vi "Read Project Path.vi"(8 "error in (no error)":errorcluster, 11 "Session in":refnum<class "Plugin Session.lvclass">) -> (0 "error out":errorcluster, 2 "Project Path":path, 3 "Session out":refnum<class "Plugin Session.lvclass">)   [LabVIEW 2021, in "InstrumentStudio Plugin SDK.lvlib" / "Plugin Session.lvclass"]
doc: "Call this VI to retrieve the absolute path of the InstrumentStudio project file on disk"
uses:
  Plugin Session.lvclass
  Plugin Session.lvclass/Plugin Session.ctl
  Read Session Id.vi
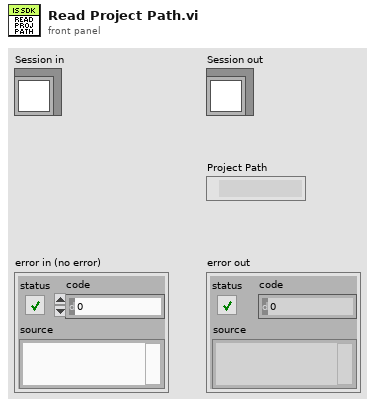
[diagram p1: front panel]
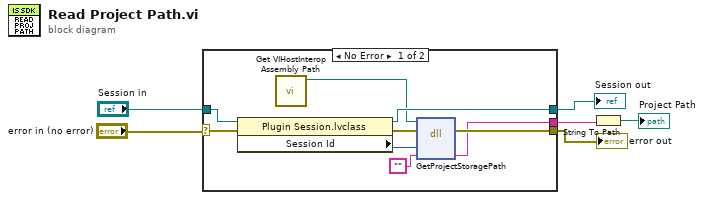
[diagram p0: block diagram]
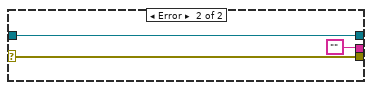
[diagram p2: hidden frame]
diagram:
  n1 = case shown="No Error" "error in (no error)" {
    selector: "error in (no error)" -> [w10 w17]
    tunnel: [w12 w17] -> w6
    tunnel: "Session in" -> [w11 w18]
    tunnel: [w9 w18] -> w3
    tunnel: [w8 ""] -> w2
    frame No Error {
      n2 = property class="Plugin Session.lvclass"(reference=w11, error in=w10) -> (reference out=w9:refnum<class "Plugin Session.lvclass">, error out=w15:errorcluster, "Session Id"=w14:u64)
      n3 = call "Get VIHostInterop Assembly Path.vi"() -> ("VIHost.Interop Assembly"=w7:path)  [unwired: 11 in]
      n4 = dll-call lib="C:/ASW/Source/InstrumentStudio/IFDistribution/VIHostPanel/objects/export/targets/win64U/x64/msvc-14.0/debug/NationalInstruments.VIHost.Interop.dll" fn="GetProjectStoragePath"(path in=w7, error in=w15, "hostId"=w14, "projectPath"="") -> (error out=w12:errorcluster, "projectPath"=w8:string)  [unwired: 3 in, 1 out]
    }
    frame Error {
    }
  }
  "error out" <- w6
  "Session out" <- w3
  n5 = String To Path(string=w2) -> (path=→"Project Path":path)
